vi "GoHome.vi"(4 "Home fail":refnum<vi>, 6 "HomeDone":refnum<vi>, 7 "Busy":refnum<vi>, 8 "error in (no error)":errorcluster, 11 "Rele in":refnum<class "Rele.lvclass">) -> (0 "error out":errorcluster, 2 "String":string, 3 "Rele out":refnum<class "Rele.lvclass">)   [LabVIEW 2012, in "Rele.lvclass"]
uses:
  Rele.lvclass
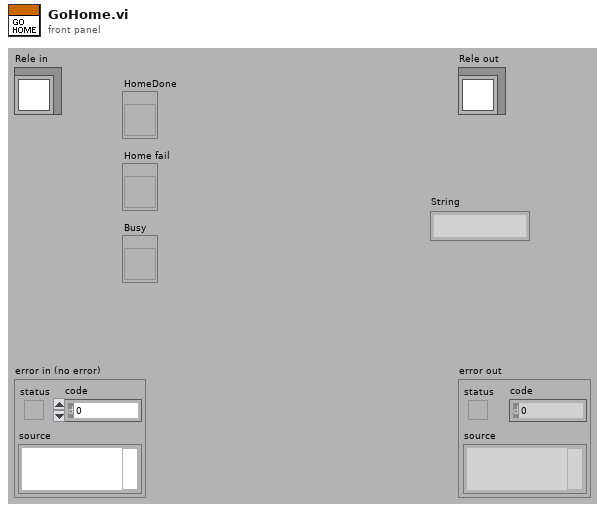
[diagram p1: front panel]
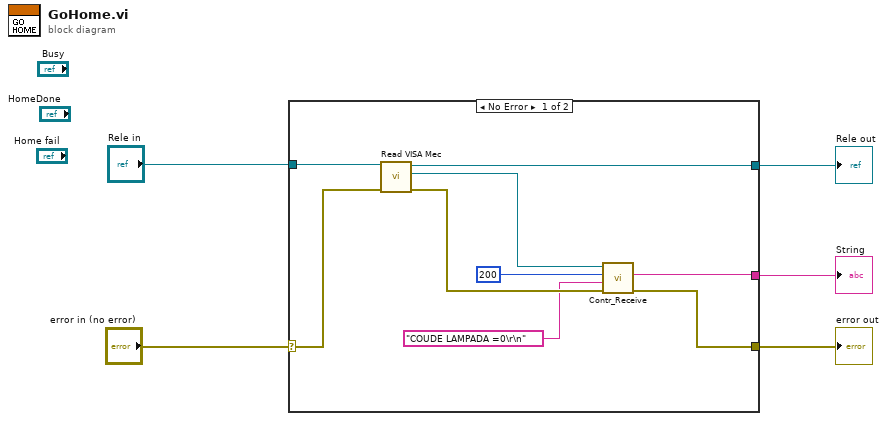
[diagram p0: block diagram]
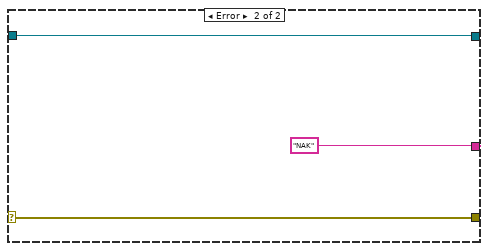
[diagram p2: hidden frame]
diagram:
  n1 = case shown="No Error" "error in (no error)" {
    selector: "error in (no error)" -> [w10 w16]
    tunnel: "Rele in" -> [w9 w17]
    tunnel: [w8 w17] -> w3
    tunnel: [w7 w16] -> w2
    tunnel: [w6 "NAK"] -> w1
    frame No Error {
      n2 = call-dynamic "Read VISA Mec.vi"("error in (no error)"=w10, "Controlador in"=w9) -> ("error out"=w14:errorcluster, "VISA Mec"=w13:refnum<visa-resource-name>, "Controlador out"=w8:refnum<class "Rele.lvclass">)  [unwired: 7 in]
      n3 = call "Contr_Receive.vi"("error in"=w14, "Command to SIFS"="COUDE LAMPADA =0\r\n", "wait after tx"=u32 200, "VISA resource name"=w13) -> ("error out"=w7:errorcluster, "Response from SIFS"=w6:string)  [unwired: 2 out]
    }
    frame Error {
    }
  }
  "error out" <- w2
  "Rele out" <- w3
  "String" <- w1
